vi "init_DAC_ao_chans.vi"(10 "Rate":dbl=80000.0 format="%#_13g") -> (0 "error out":errorcluster, 2 "Actual Sample Rate":dbl=1000.0 format="%0.2f", 3 "Refnum out":refnum<k21>)   [LabVIEW 2015]
uses:
  <vilib>/DAQmx/create/channels.llb/DAQmx Create Channel (AO-Voltage-Basic).vi
  <vilib>/DAQmx/configure/timing.llb/DAQmx Timing (Sample Clock).vi
  <resource>/objmgr/daqmx.rc
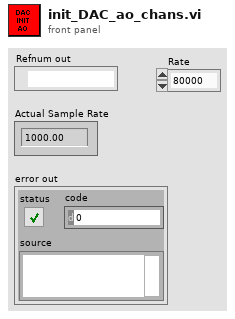
[diagram p1: front panel]
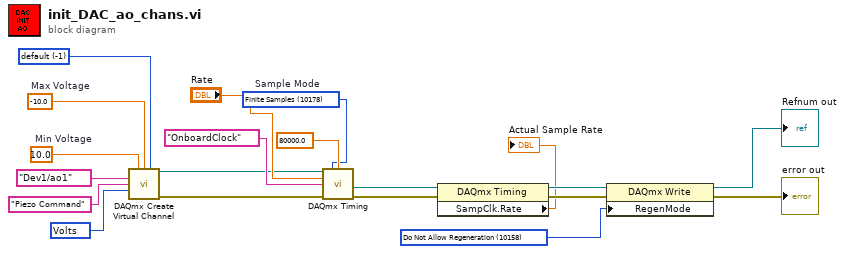
[diagram p0: block diagram]
diagram:
  w20 = 10158 items=["Allow Regeneration"=10097, "Do Not Allow Regeneration"=10158] ("RegenMode")
  w10 = 10178 items=["Finite Samples"=10178, "Continuous Samples"=10123, "Hardware Timed Single Point"=12522]  # Sample Mode
  w9 = -1 items=["default"=-1, "RSE"=10083, "NRSE"=10078, "Differential"=10106, "Pseudodifferential"=12529] ("input terminal configuration")
  w8 = 10348 items=["Volts"=10348, "From Custom Scale"=10065] ("units")
  w4 = 10.0  # Min Voltage
  w5 = -10.0  # Max Voltage
  n1 = call-poly <vilib>:"DAQmx Create Virtual Channel.vi"("maximum value"=w4, "minimum value"=w5, "output terminal configuration"=w9, "physical channels"=tag "Dev1/ao1" ("DAQmx Physical Channel"), "name to assign"="Piezo Command", "units"=w8) -> ("task out"=w2:refnum<k21>, "error out"=w1:errorcluster)  [unwired: 8 in]
  n2 = call-poly <vilib>:"DAQmx Timing.vi"("task/channels in"=w2, "sample mode"=w10, "samples per channel"=80000.0, "rate"="Rate", "source"=tag "OnboardClock" ("Sample Clock Source"), "error in"=w1) -> ("task out"=w12:refnum<k21>, "error out"=w13:errorcluster)  [unwired: 8 in]
  n3 = property class="DAQmx Timing"(reference=w12, error in=w13) -> (reference out=w16:refnum<k21>, error out=w17:errorcluster, "SampClk.Rate"=→"Actual Sample Rate":dbl)
  n4 = property class="DAQmx Write"(reference=w16, error in=w17, "RegenMode"=w20) -> (reference out=→"Refnum out":refnum<k21>, error out=→"error out":errorcluster)
